vi "Referect_EnableCh_for_form.vi"(8 "错误输入（无错误）":errorcluster, 10 "MPM":refnum<k24>[](array[refnum]), 11 "数组输入":bool[](array[boolean])) -> (0 "error IO":errorcluster, 3 "数组输出":bool[](array[boolean]))   [LabVIEW 2017]
uses:
  D:/test/ILSTS/LV_IL_Sample/DLL/InstrumentDLL.dll
  DLL/InstrumentDLL.dll
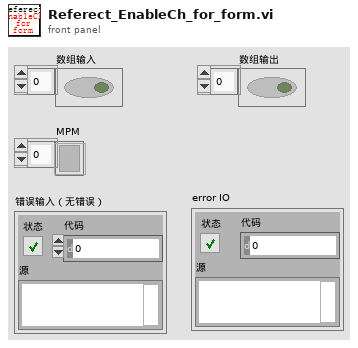
[diagram p1: front panel]
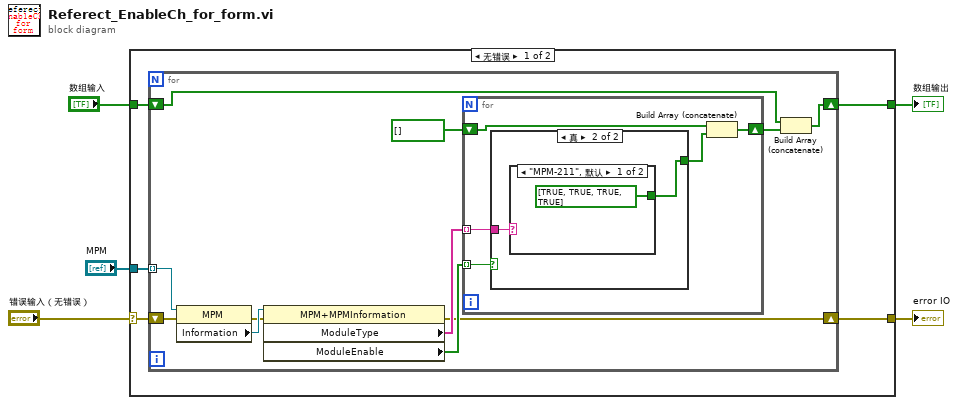
[diagram p0: block diagram]
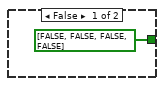
[diagram p2: hidden frame]
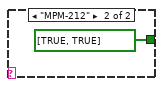
[diagram p3: hidden frame]
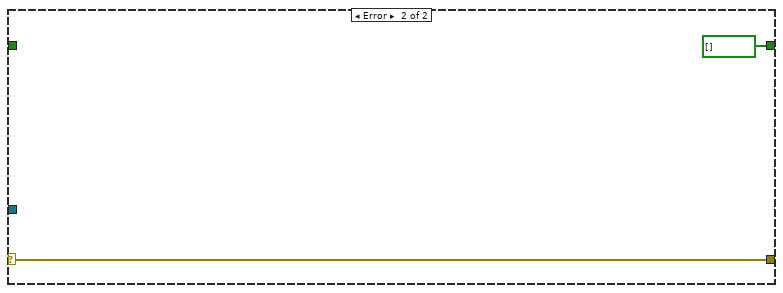
[diagram p4: hidden frame]
diagram:
  n1 = case shown="无错误" "错误输入（无错误）" {
    selector: "错误输入（无错误）" -> [w7 w32]
    tunnel: [w10 bool[] [] ("数组输入")] -> w5
    tunnel: "数组输入" -> [w9 _]
    tunnel: "MPM" -> [w8 _]
    tunnel: [w6 w32] -> w1
    frame No Error {
      n2 = for {
        tunnel: w8 -> [w20] mode=indexing
        shift-right: [w14] -> w10
        shift-left: w9 -> [w18]
        shift-right: [w11] -> w6
        shift-left: w7 -> [w13]
        n3 = property on="属性节点" class="MPM"(reference=w20, error in=w13) -> (error out=w12:errorcluster, "Information"=w21:refnum<k24>)  [unwired: 1 out]
        n4 = property class="MPM+MPMInformation"(reference=w21, error in=w12) -> (error out=w11:errorcluster, "ModuleType"=w19:string[], "ModuleEnable"=w15:bool[])  [unwired: 1 out]
        n5 = for {
          tunnel: w19 -> [w26] mode=indexing
          shift-right: [w23] -> w16
          shift-left: bool[] [] ("添加的数组") -> [w24]
          tunnel: w15 -> [w22] mode=indexing
          n6 = case shown="真" w22 {
            tunnel: w26 -> [_ w29]
            tunnel: [bool[] [FALSE, FALSE, FALSE, FALSE] w28] -> w25
            frame False {
            }
            frame True {
              n7 = case shown="\"MPM-211\", 默认" w29 {
                tunnel: [bool[] [TRUE, TRUE, TRUE, TRUE] bool[] [TRUE, TRUE]] -> w28
                frame "MPM-211", Default {
                }
                frame "MPM-212" {
                }
              }
            }
          }
          n8 = Build Array (concatenate)(w24, w25) -> (w23:bool[])
        }
        n9 = Build Array (concatenate)(w18, w16) -> (w14:bool[])
      }
    }
    frame Error {
    }
  }
  "数组输出" <- w5
  "error IO" <- w1
